vi "spy satellite.vi"() -> ()   [LabVIEW 2012]
uses:
  <vilib>/imath/engines/lvmath2/RunTimeEngine/NodeEndStatement/NIMS_NodeEndStatement_Output.vi
  <instcachedir>/0/NIMS_NodeEndStatement_Output_53EC0D466D134D7ABD903AC30B43404B.lvgen/NIMS_NodeEndStatement_Output_53EC0D466D134D7ABD903AC30B43404B_001.vi
  <vilib>/imath/engines/lvmath2/RunTimeEngine/ErrorHandling/NIMS_Finalize Error.vi
  <vilib>/imath/engines/lvmath2/RunTimeEngine/ReplaceToken/NIMS_Replace - Check Row.vi
  <instcachedir>/0/NIMS_Replace - Check Row_8C35B66FE73A429EAC382AAA935851F0.lvgen/NIMS_Replace - Check Row_8C35B66FE73A429EAC382AAA935851F0_005.vi
  <vilib>/imath/engines/lvmath2/RunTimeEngine/ReplaceToken/NIMS_Replace - Check Column.vi
  <instcachedir>/0/NIMS_Replace - Check Column_F9ADE87E459D46779ACFAE3AFB317B9B.lvgen/NIMS_Replace - Check Column_F9ADE87E459D46779ACFAE3AFB317B9B_007.vi
  <vilib>/imath/engines/lvmath2/RunTimeEngine/BuiltInFunctions/size/NIMS_I32=size(GRow,I32).vi
  <instcachedir>/0/NIMS_I32=size(GRow,I32)_2314177FB7B742BE809A342F8CD00E1F.lvgen/NIMS_I32=size(GRow,I32)_2314177FB7B742BE809A342F8CD00E1F_000.vi
  <vilib>/imath/engines/lvmath2/RunTimeEngine/ReplaceToken/NIMS_Replace - Size Check M(_,_)=S.vi
  <instcachedir>/0/NIMS_Replace - Size Check M(_,_)=S_0CFA00F12BB840EDA61E43D782562782.lvgen/NIMS_Replace - Size Check M(_,_)=S_0CFA00F12BB840EDA61E43D782562782_002.vi
  <vilib>/imath/engines/lvmath2/RunTimeEngine/ReplaceToken/NIMS_Replace - M(S,S)=S.vi
  <instcachedir>/0/NIMS_Replace - M(S,S)=S_59120E3D3E804D63A1B2B7FDD4B95F55.lvgen/NIMS_Replace - M(S,S)=S_59120E3D3E804D63A1B2B7FDD4B95F55_002.vi
  <vilib>/imath/engines/lvmath2/RunTimeEngine/ErrorHandling/NIMS_Create Error From Enums.vi
  <instcachedir>/0/NIMS_I32=size(GRow,I32)_2314177FB7B742BE809A342F8CD00E1F.lvgen/NIMS_I32=size(GRow,I32)_2314177FB7B742BE809A342F8CD00E1F_001.vi
  <vilib>/imath/engines/lvmath2/RunTimeEngine/BuiltInFunctions/size/NIMS_I32=size(GM,I32).vi
  <instcachedir>/0/NIMS_I32=size(GM,I32)_AF436776B5724EA8A5CFD6FACA63D3D9.lvgen/NIMS_I32=size(GM,I32)_AF436776B5724EA8A5CFD6FACA63D3D9_004.vi
  <instcachedir>/0/NIMS_NodeEndStatement_Output_53EC0D466D134D7ABD903AC30B43404B.lvgen/NIMS_NodeEndStatement_Output_53EC0D466D134D7ABD903AC30B43404B_003.vi
  <vilib>/imathl/engines/lvmath/Functions/Error Handling/Create Error.vi
  <vilib>/imath/engines/lvmath2/RunTimeEngine/VariableToken/Read/NIMS_Get Elements - SorM(_,_) - Check - Check.vi
  <instcachedir>/0/NIMS_Get Elements - SorM(_,_) - Check - Check_3492346BAECA4EC09E2016EA7EC0034B.lvgen/NIMS_Get Elements - SorM(_,_) - Check - Check_3492346BAECA4EC09E2016EA7EC0034B_006.vi
  <instcachedir>/0/NIMS_Replace - Check Row_8C35B66FE73A429EAC382AAA935851F0.lvgen/NIMS_Replace - Check Row_8C35B66FE73A429EAC382AAA935851F0_007.vi
  <instcachedir>/0/NIMS_Replace - Check Column_F9ADE87E459D46779ACFAE3AFB317B9B.lvgen/NIMS_Replace - Check Column_F9ADE87E459D46779ACFAE3AFB317B9B_008.vi
  <vilib>/imath/engines/lvmath2/RunTimeEngine/VariableToken/Read/NIMS_Get Elements - RV(_,_) - Check - Check.vi
  <instcachedir>/0/NIMS_Get Elements - RV(_,_) - Check - Check_2E99379E6D1246468E5A333FCE5C48DF.lvgen/NIMS_Get Elements - RV(_,_) - Check - Check_2E99379E6D1246468E5A333FCE5C48DF_000.vi
  <instcachedir>/0/NIMS_Replace - Size Check M(_,_)=S_0CFA00F12BB840EDA61E43D782562782.lvgen/NIMS_Replace - Size Check M(_,_)=S_0CFA00F12BB840EDA61E43D782562782_003.vi
  <instcachedir>/0/NIMS_Replace - M(S,S)=S_59120E3D3E804D63A1B2B7FDD4B95F55.lvgen/NIMS_Replace - M(S,S)=S_59120E3D3E804D63A1B2B7FDD4B95F55_003.vi
  <instcachedir>/0/NIMS_Replace - Check Row_8C35B66FE73A429EAC382AAA935851F0.lvgen/NIMS_Replace - Check Row_8C35B66FE73A429EAC382AAA935851F0_000.vi
  <instcachedir>/0/NIMS_Replace - Check Column_F9ADE87E459D46779ACFAE3AFB317B9B.lvgen/NIMS_Replace - Check Column_F9ADE87E459D46779ACFAE3AFB317B9B_001.vi
  <instcachedir>/0/NIMS_Get Elements - RV(_,_) - Check - Check_2E99379E6D1246468E5A333FCE5C48DF.lvgen/NIMS_Get Elements - RV(_,_) - Check - Check_2E99379E6D1246468E5A333FCE5C48DF_001.vi
  <instcachedir>/0/NIMS_Replace - Size Check M(_,_)=S_0CFA00F12BB840EDA61E43D782562782.lvgen/NIMS_Replace - Size Check M(_,_)=S_0CFA00F12BB840EDA61E43D782562782_000.vi
  <instcachedir>/0/NIMS_Replace - M(S,S)=S_59120E3D3E804D63A1B2B7FDD4B95F55.lvgen/NIMS_Replace - M(S,S)=S_59120E3D3E804D63A1B2B7FDD4B95F55_000.vi
  <instcachedir>/0/NIMS_Get Elements - SorM(_,_) - Check - Check_3492346BAECA4EC09E2016EA7EC0034B.lvgen/NIMS_Get Elements - SorM(_,_) - Check - Check_3492346BAECA4EC09E2016EA7EC0034B_001.vi
  <vilib>/imath/engines/lvmath2/RunTimeEngine/RangeToken/NIMS_Range_R2 - Integer.vi
  <instcachedir>/0/NIMS_Range_R2 - Integer_CD92A44154CA48D58B2F3E711AB114DB.lvgen/NIMS_Range_R2 - Integer_CD92A44154CA48D58B2F3E711AB114DB_000.vi
  <vilib>/imath/engines/lvmath2/RunTimeEngine/CommandStatement/MC_CommandStatement_break.vi
  <vilib>/imath/engines/lvmath2/RunTimeEngine/BuiltInFunctions/asin/NIMS_asin(C).vi
  <instcachedir>/0/NIMS_asin(C)_F3E14D7F5FA648E9BF65D5738488DD5F.lvgen/NIMS_asin(C)_F3E14D7F5FA648E9BF65D5738488DD5F_001.vi
  <vilib>/imath/engines/lvmath2/RunTimeEngine/BuiltInFunctions/cos/NIMS_cos(C).vi
  <instcachedir>/0/NIMS_cos(C)_41CCDEE9AC714B93BD437808B3FF118A.lvgen/NIMS_cos(C)_41CCDEE9AC714B93BD437808B3FF118A_001.vi
  <vilib>/imath/engines/lvmath2/RunTimeEngine/BuiltInFunctions/round/NIMS_round(CDB-S).vi
  <vilib>/imath/engines/lvmath2/RunTimeEngine/VariableToken/NIMS_VariableToken_CondDefinedDefinedByReplace.vi
  <instcachedir>/0/NIMS_VariableToken_CondDefinedDefinedByReplace_D162CFFC24174562A9FEA619A91E1A56.lvgen/NIMS_VariableToken_CondDefinedDefinedByReplace_D162CFFC24174562A9FEA619A91E1A56_002.vi
  <instcachedir>/0/NIMS_Replace - Check Row_8C35B66FE73A429EAC382AAA935851F0.lvgen/NIMS_Replace - Check Row_8C35B66FE73A429EAC382AAA935851F0_006.vi
  <instcachedir>/0/NIMS_Replace - Check Column_F9ADE87E459D46779ACFAE3AFB317B9B.lvgen/NIMS_Replace - Check Column_F9ADE87E459D46779ACFAE3AFB317B9B_003.vi
  <instcachedir>/0/NIMS_Replace - Size Check M(_,_)=S_0CFA00F12BB840EDA61E43D782562782.lvgen/NIMS_Replace - Size Check M(_,_)=S_0CFA00F12BB840EDA61E43D782562782_001.vi
  <instcachedir>/0/NIMS_Replace - M(S,S)=S_59120E3D3E804D63A1B2B7FDD4B95F55.lvgen/NIMS_Replace - M(S,S)=S_59120E3D3E804D63A1B2B7FDD4B95F55_001.vi
  <vilib>/imath/engines/lvmath2/RunTimeEngine/VariableToken/NIMS_VariableToken_CondDefined.vi
  <instcachedir>/0/NIMS_VariableToken_CondDefined_295AAB8C64C949DA8EA45AB7820AF759.lvgen/NIMS_VariableToken_CondDefined_295AAB8C64C949DA8EA45AB7820AF759_002.vi
  <instcachedir>/0/NIMS_Get Elements - SorM(_,_) - Check - Check_3492346BAECA4EC09E2016EA7EC0034B.lvgen/NIMS_Get Elements - SorM(_,_) - Check - Check_3492346BAECA4EC09E2016EA7EC0034B_007.vi
  <vilib>/imath/engines/lvmath2/RunTimeEngine/BuiltInFunctions/atan2/NIMS_atan2.vi
  <instcachedir>/0/NIMS_atan2_A91AA4A7D42247EDBE8F76DB99AF04A4.lvgen/NIMS_atan2_A91AA4A7D42247EDBE8F76DB99AF04A4_000.vi
panel:
  out "Angle 1":sgl
  out "Tank1":T1(array[cluster]) {"Bounding Box"."y" format="%.2f"; "Bounding Box"."x" format="%.2f"; "Position"."y" format="%.2f"; "Position"."x" format="%.2f"; "Score" format="%.2f"; "Scale" format="%.2f"; "Angle" format="%.2f"}
  out "Tank2":T1(array[cluster]) {"Bounding Box"."y" format="%.2f"; "Bounding Box"."x" format="%.2f"; "Position"."y" format="%.2f"; "Position"."x" format="%.2f"; "Score" format="%.2f"; "Scale" format="%.2f"; "Angle" format="%.2f"}
  out "Angle 2":sgl
  out "Ball":dbl[][](array[numeric])
  out "Image 3":T2(plugin-control)
  out "direction2":dbl
  out "direction1":dbl
  out "Ball":dbl[][](array[numeric]) format="%.2f"
  out "Tank2":dbl[][](array[numeric]) format="%.2f"
  out "Tank1":dbl[][](array[numeric]) format="%.2f"
  in  "Stop (F)":bool
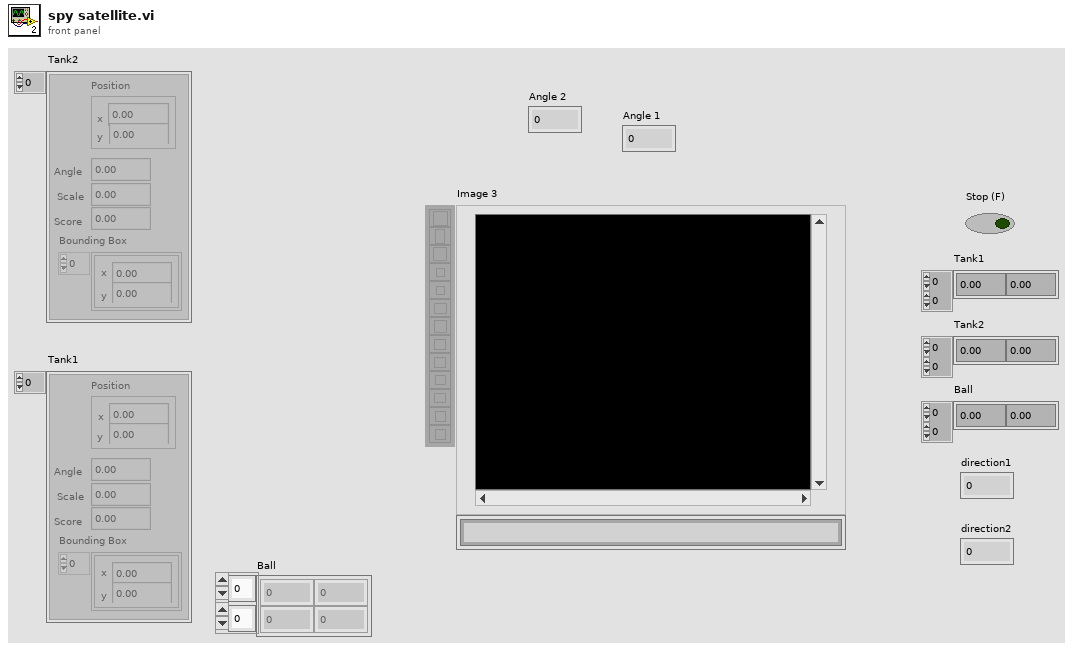
[diagram p1: front panel]
types:
  T1 = cluster{"Position":cluster{"x":sgl, "y":sgl}, "Angle":sgl, "Scale":sgl, "Score":sgl, "Bounding Box":cluster{"x":sgl, "y":sgl}[]}[]
  T2 = typedef "IMAQ Image.ctl" = refnum<image>
  T3 = typedef "Image Type" = u32
  T4 = cluster{"Position":cluster{"x":sgl, "y":sgl}, "Angle":sgl, "Scale":sgl, "Score":sgl, "Bounding Box":cluster{"x":sgl, "y":sgl}[]}
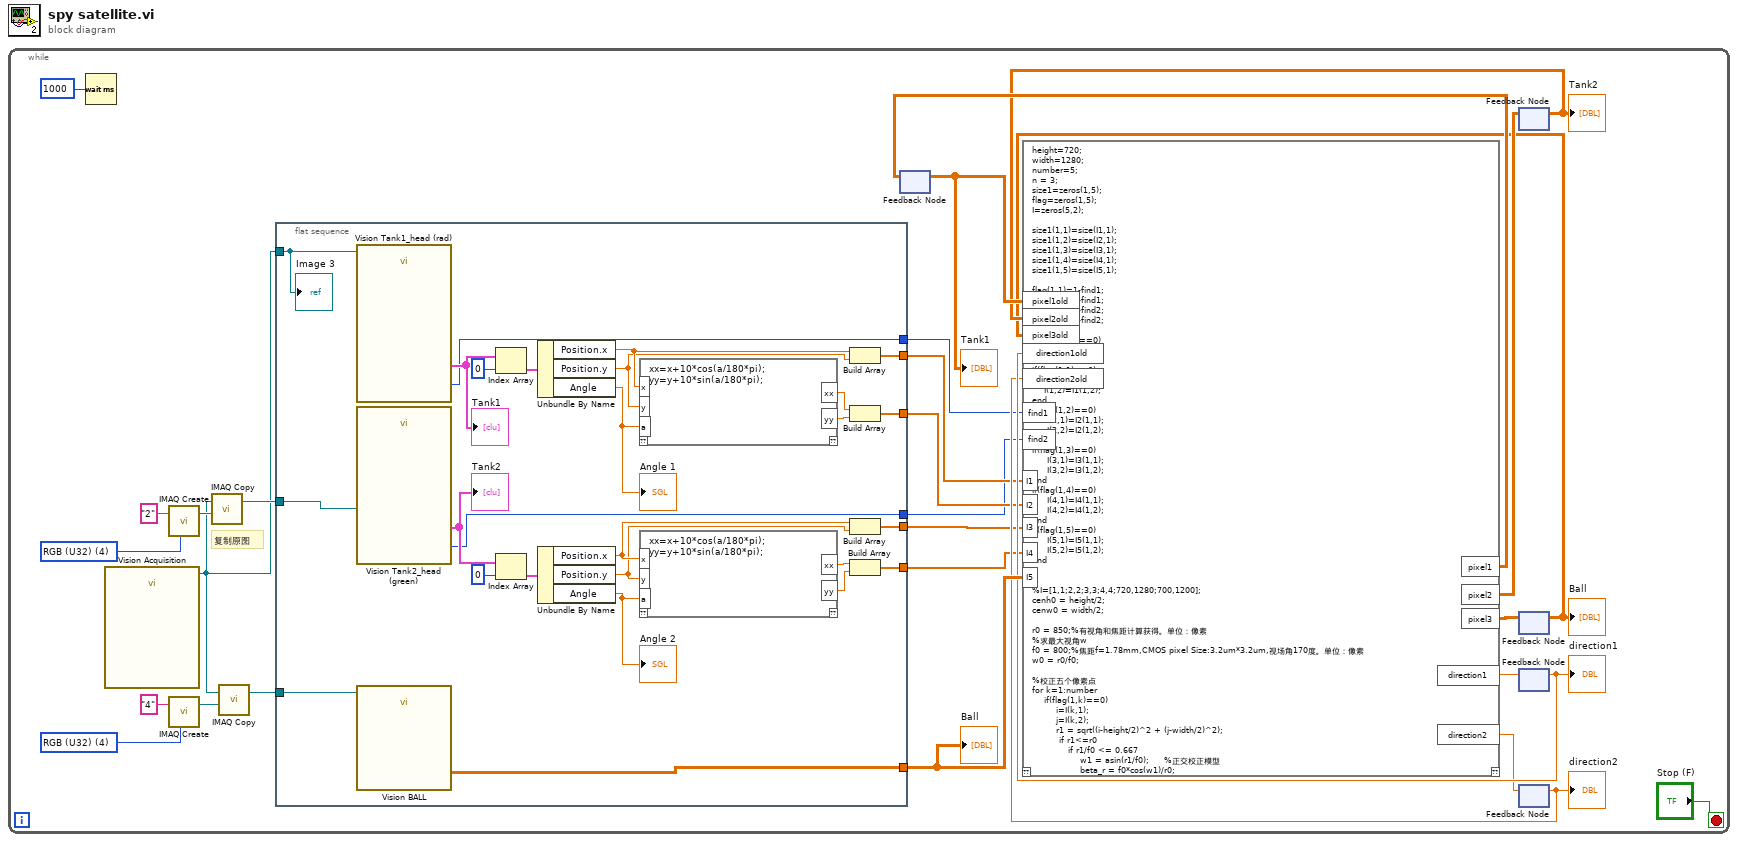
[diagram p0: block diagram]
diagram:
  n1 = while {
    stop <- "Stop (F)" stop-if-true
    w20 = T3 4 items=["Grayscale (U8)", "Grayscale (I16)", "Grayscale (SGL)", "Complex (CSG)", "RGB (U32)", "HSL (U32)", "RGB (U64)", "Grayscale (U16)"] ("Image Type")
    w24 = T3 4 items=["Grayscale (U8)", "Grayscale (I16)", "Grayscale (SGL)", "Complex (CSG)", "RGB (U32)", "HSL (U32)", "RGB (U64)", "Grayscale (U16)"] ("Image Type")
    # "复制原图"
    n2 = Wait (ms)(milliseconds to wait=u32 1000) -> ()  [unwired: 1 out]
    n3 = call "Vision Acquisition"() -> ("Image Out"=w18:T2)  [unwired: 26 in, 1 out]
    n4 = call "IMAQ Create"("Image Name"="2", "Image Type"=w24) -> ("New Image"=w25:T2)  [unwired: 3 in, 1 out]
    n5 = call "IMAQ Create"("Image Name"="4", "Image Type"=w20) -> ("New Image"=w21:T2)  [unwired: 3 in, 1 out]
    n6 = call "IMAQ Copy"("Image Dst"=w25, "Image Src"=w18) -> ("Image Dst Out"=w23:T2)  [unwired: 4 in, 1 out]
    n7 = call "IMAQ Copy"("Image Dst"=w21, "Image Src"=w18) -> ("Image Dst Out"=w19:T2)  [unwired: 4 in, 1 out]
    n8 = flat-sequence {
      tunnel: w18 -> [w54]
      tunnel: w23 -> [w53]
      tunnel: w19 -> [w52]
      tunnel: [w51] -> w17
      tunnel: [w47] -> w6
      tunnel: [w43] -> w5
      tunnel: [w42] -> w4
      tunnel: [w33] -> w3
      tunnel: [w30] -> w2
      tunnel: [w29] -> w1
      frame #0 {
        n9 = call "Vision Tank1_head (rad)"("Image In"=w54) -> ("Matches (Pattern Matching 1)"=w44:T1, "Number of Matches (Pattern Matching 1)"=w29:i32)  [unwired: 23 in, 2 out]
        "Tank1" <- w44
        n10 = call "Vision Tank2_head (green)"("Image In"=w53) -> ("Matches (Pattern Matching 1)"=w50:T1, "Number of Matches (Pattern Matching 1)"=w30:i32)  [unwired: 23 in, 2 out]
        "Tank2" <- w50
        n11 = call "Vision BALL"("Image In"=w52) -> ("Particle Measurements (Pixels) (Particle Analysis 1)"=w51:dbl[][])  [unwired: 23 in, 3 out]
        n12 = Index Array(array=w44, index=0) -> (element=w45:T4)
        n13 = Index Array(array=w50, index=0) -> (element=w48:T4)
        n14 = Unbundle By Name(w45) -> ("Position.x"=w41:sgl, "Position.y"=w40:sgl, "Angle"=w39:sgl)
        "Angle 1" <- w39
        n15 = Unbundle By Name(w48) -> ("Position.x"=w36:sgl, "Position.y"=w35:sgl, "Angle"=w34:sgl)
        "Angle 2" <- w34
        n16 = mathscript code="xx=x+10*cos(a/180*pi);\nyy=y+10*sin(a/180*pi);"("x"=w41, "y"=w40, "a"=w39) -> ("xx"=w38:dbl, "yy"=w37:dbl)  [unwired: 1 in, 1 out]
        n17 = mathscript code="xx=x+10*cos(a/180*pi);\nyy=y+10*sin(a/180*pi);"("x"=w36, "y"=w35, "a"=w34) -> ("xx"=w32:dbl, "yy"=w31:dbl)  [unwired: 1 in, 1 out]
        n18 = Build Array(w41, w40) -> (w43:sgl[])
        n19 = Build Array(w38, w37) -> (w42:dbl[])
        n20 = Build Array(w36, w35) -> (w47:sgl[])
        n21 = Build Array(w32, w31) -> (w33:dbl[])
        "Image 3" <- w54
      }
    }
    n22 = feedback #1() -> (w15:cdb[][])  [unwired: 1 in]
    "Tank1" <- w15
    n23 = feedback #2() -> (w13:cdb[][])  [unwired: 1 in]
    "Tank2" <- w13
    n24 = feedback #3() -> (w11:cdb[][])  [unwired: 1 in]
    "Ball" <- w11
    n25 = feedback #4() -> (w9:dbl)  [unwired: 1 in]
    "direction1" <- w9
    n26 = feedback #5() -> (w7:dbl)  [unwired: 1 in]
    "direction2" <- w7
    n27 = mathscript code="height=720;\nwidth=1280;\nnumber=5;\nn = 3;\nsize1=zeros(1,5);\nflag=zeros(1,5);\nI=zeros(5,2);\n\nsize1(1,1)=size(I1,1);\nsize1(1,2)=size(I2,1);\nsize1(1,3)=size(I3,1);\nsize1(1,4)=size(I4,1);\nsize1(1,5)=size(I5,1);\n\nflag(1,1)=1-find1;\nflag(1,2)=1-find1;\nflag(1,3)=1-find2;\nflag(1,4)=1-find2;\n\nif(size1(1,5)==0)\n    flag(1,5)=1;\nend\nif(flag(1,1)==0)\n    I(1,1)=I1(1,1);\n    I(1,2)=I1(1,2);\nend\nif(flag(1,2)==0)\n     I(2,1)=I2(1,1);\n     I(2,2)=I2(1,2);\nend\nif(flag(1,3)==0)\n     I(3,1)=I3(1,1);\n     I(3,2)=I3(1,2);\nend\nif(flag(1,4)==0)\n     I(4,1)=I4(1,1);\n     I(4,2)=I4(1,2);\nend\nif(flag(1,5)==0)\n     I(5,1)=I5(1,1);\n     I(5,2)=I5(1,2);\nend\n\n\n%I=[1,1;2,2;3,3;4,4;720,1280;700,1200];\ncenh0 = height/2;\ncenw0 = width/2;\n\nr0 = 850;%有视角和焦距计算获得。单位：像素\n%求最大视角w\nf0 = 800;%焦距f=1.78mm,CMOS pixel Size:3.2um*3.2um,视场角170度。单位：像素\nw0 = r0/f0;\n\n%校正五个像素点\nfor k=1:number\n    if(flag(1,k)==0)\n        i=I(k,1);\n        j=I(k,2);\n        r1 = sqrt((i-height/2)^2 + (j-width/2)^2);\n         if r1<=r0\n            if r1/f0 <= 0.667\n                w1 = asin(r1/f0);     %正交校正模型\n                beta_r = f0*cos(w1)/r0;\n                 \n            elseif r1/f0 <= 0.78           %2*f0\n                w1 = 2*asin(r1/f0/2); %等立体角修正模型\n                beta_r = f0*cos(w1/2)/r0;\n            else\n                w1 = r0/f0;           %等距修正模型\n               beta_r = f0/r0;\n             end\n        else\n            beta_r = 0.000001;\n        end\n        x = height*n/2 + (i-cenh0)/beta_r;\n        y = width*n/2 + (j-cenw0)/beta_r;     \n        x = round(x);\n        y = round(y);\n \n%         if (x>0) && (x<n*height) && (y>0) && (y<n*width)\n        IR(k,1)=x;\n        IR(k,2)=y;\n%         end\n    end\nend\n%根据抓取情况更新数据\nif(flag(1,1)==0&&flag(1,2)==0)\n    direction1=atan2(IR(1,2)-IR(2,2),IR(1,1)-IR(2,1));\n    pixel1(1,1)=IR(1,1)/2/135*0.6-6.83;\n    pixel1(1,2)=IR(1,2)/2/135*0.6-7.2;\nelse\n    pixel1=pixel1old;\n    direction1=direction1old;\nend\n\nif(flag(1,3)==0&&flag(1,4)==0)\n    direction2=atan2(IR(3,2)-IR(4,2),IR(3,1)-IR(4,1));\n    pixel2(1,1)=IR(3,1)/2/135*0.6-6.83;\n    pixel2(1,2)=IR(3,2)/2/135*0.6-7.2;\nelse\n    pixel2=pixel2old;\n    direction2=direction2old;\nend\nif(flag(1,5)==0)\n    pixel3(1,1)=IR(5,1)/135*0.6-6.83;\n    pixel3(1,2)=IR(5,2)/135*0.6-7.2;\nelse\n    pixel3=pixel3old;\nend\n\n% hold on\n% if(flag(1,5)==0)\n% scatter(pixel3(1,1),pixel3(1,2));\n% end"("I1"=w5, "I2"=w4, "I3"=w6, "I4"=w3, "I5"=w17, "pixel1old"=w15, "pixel2old"=w13, "pixel3old"=w11, "direction1old"=w9, "direction2old"=w7, "find1"=w1, "find2"=w2) -> ("pixel1"=w16:cdb[][], "pixel2"=w14:cdb[][], "pixel3"=w12:cdb[][], "direction1"=w10:dbl, "direction2"=w8:dbl)  [unwired: 1 in, 1 out]
    n28 = feedback-in #1(w16) -> ()
    n29 = feedback-in #2(w14) -> ()
    n30 = feedback-in #3(w12) -> ()
    n31 = feedback-in #4(w10) -> ()
    n32 = feedback-in #5(w8) -> ()
    "Ball" <- w17
  }
